vi "test-Implicit-Model-Follower-Test1.vi"(8 "error in (no error)":errorcluster) -> (0 "error out":errorcluster, 3 "All tests passed":bool)   [LabVIEW 2019]
uses:
  <vilib>/Rock Robotics/WPI/ThirdParty/JAS_Junk/TrajLib/MatBuilder_Create.vi
  <vilib>/Rock Robotics/WPI/ThirdParty/JAS_Junk/TrajLib/LinearSystem_New.vi
  <vilib>/Rock Robotics/WPI/ThirdParty/JAS_Junk/TrajLib/MatrixHelper_Zero.vi
  <vilib>/Rock Robotics/WPI/ThirdParty/JAS_Junk/TrajLib/Discretization_DiscretizeAB.vi
  <vilib>/Analysis/baseanly.llb/A x B.vi
  <vilib>/Analysis/baseanly.llb/Real A x B.vi
  <vilib>/Rock Robotics/WPI/ThirdParty/JAS_Junk/TrajLib/MatrixHelper_CoerceSize.vi
  <vilib>/Rock Robotics/WPI/ThirdParty/JAS_Junk/TrajLib/Matrix_Exp.vi
  <vilib>/Rock Robotics/WPI/ThirdParty/JAS_Junk/TrajLib/Matrix_AssignBlock.vi
  <vilib>/Rock Robotics/WPI/ThirdParty/JAS_Junk/TrajLib/Matrix_ExtractFrom.vi
  <vilib>/Analysis/7linalg.llb/Matrix Exp.vi
  <vilib>/Analysis/7linalg.llb/Real Matrix Exp.vi
  <vilib>/Analysis/Matrix/Numeric/Multiply/Multiply.vi
  <vilib>/Analysis/Matrix/Numeric/Multiply/Multiply - RM,R.vi
  <vilib>/Analysis/Matrix/Numeric/Add/Add.vi
  <vilib>/Analysis/Matrix/Numeric/Add/Add - RM,RM.vi
  <vilib>/Rock Robotics/WPI/ThirdParty/JAS_Junk/TrajLib/Trajectory_Library.lvlib
panel:
  out "Test 3":bool
  out "Test 2":bool
  out "Test 1":bool
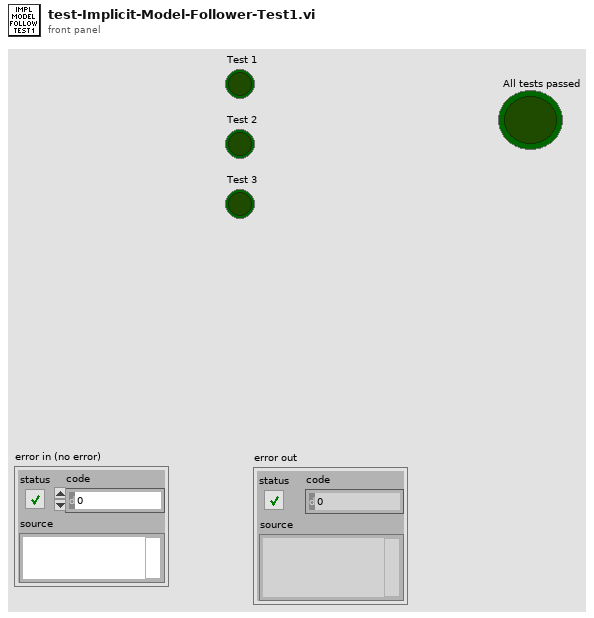
[diagram p1: front panel]
types:
  T1 = typedef "NI_Matrix.lvlib/RealMatrix.ctl" = dbl[][]
  T2 = typedef "Trajectory_Library.lvlib/LINEAR_SYSTEM.ctl" = cluster{"m_A":T1, "m_B":T1, "m_C":T1, "m_D":T1, "States":i32, "Inputs":i32, "Outputs":i32}
  T3 = typedef "Trajectory_Library.lvlib/IMPLICIT_MODEL_FOLLOWER.ctl" = cluster{"m_A":T1, "m_B":T1, "m_U":T1, "States":i32, "Inputs":i32}
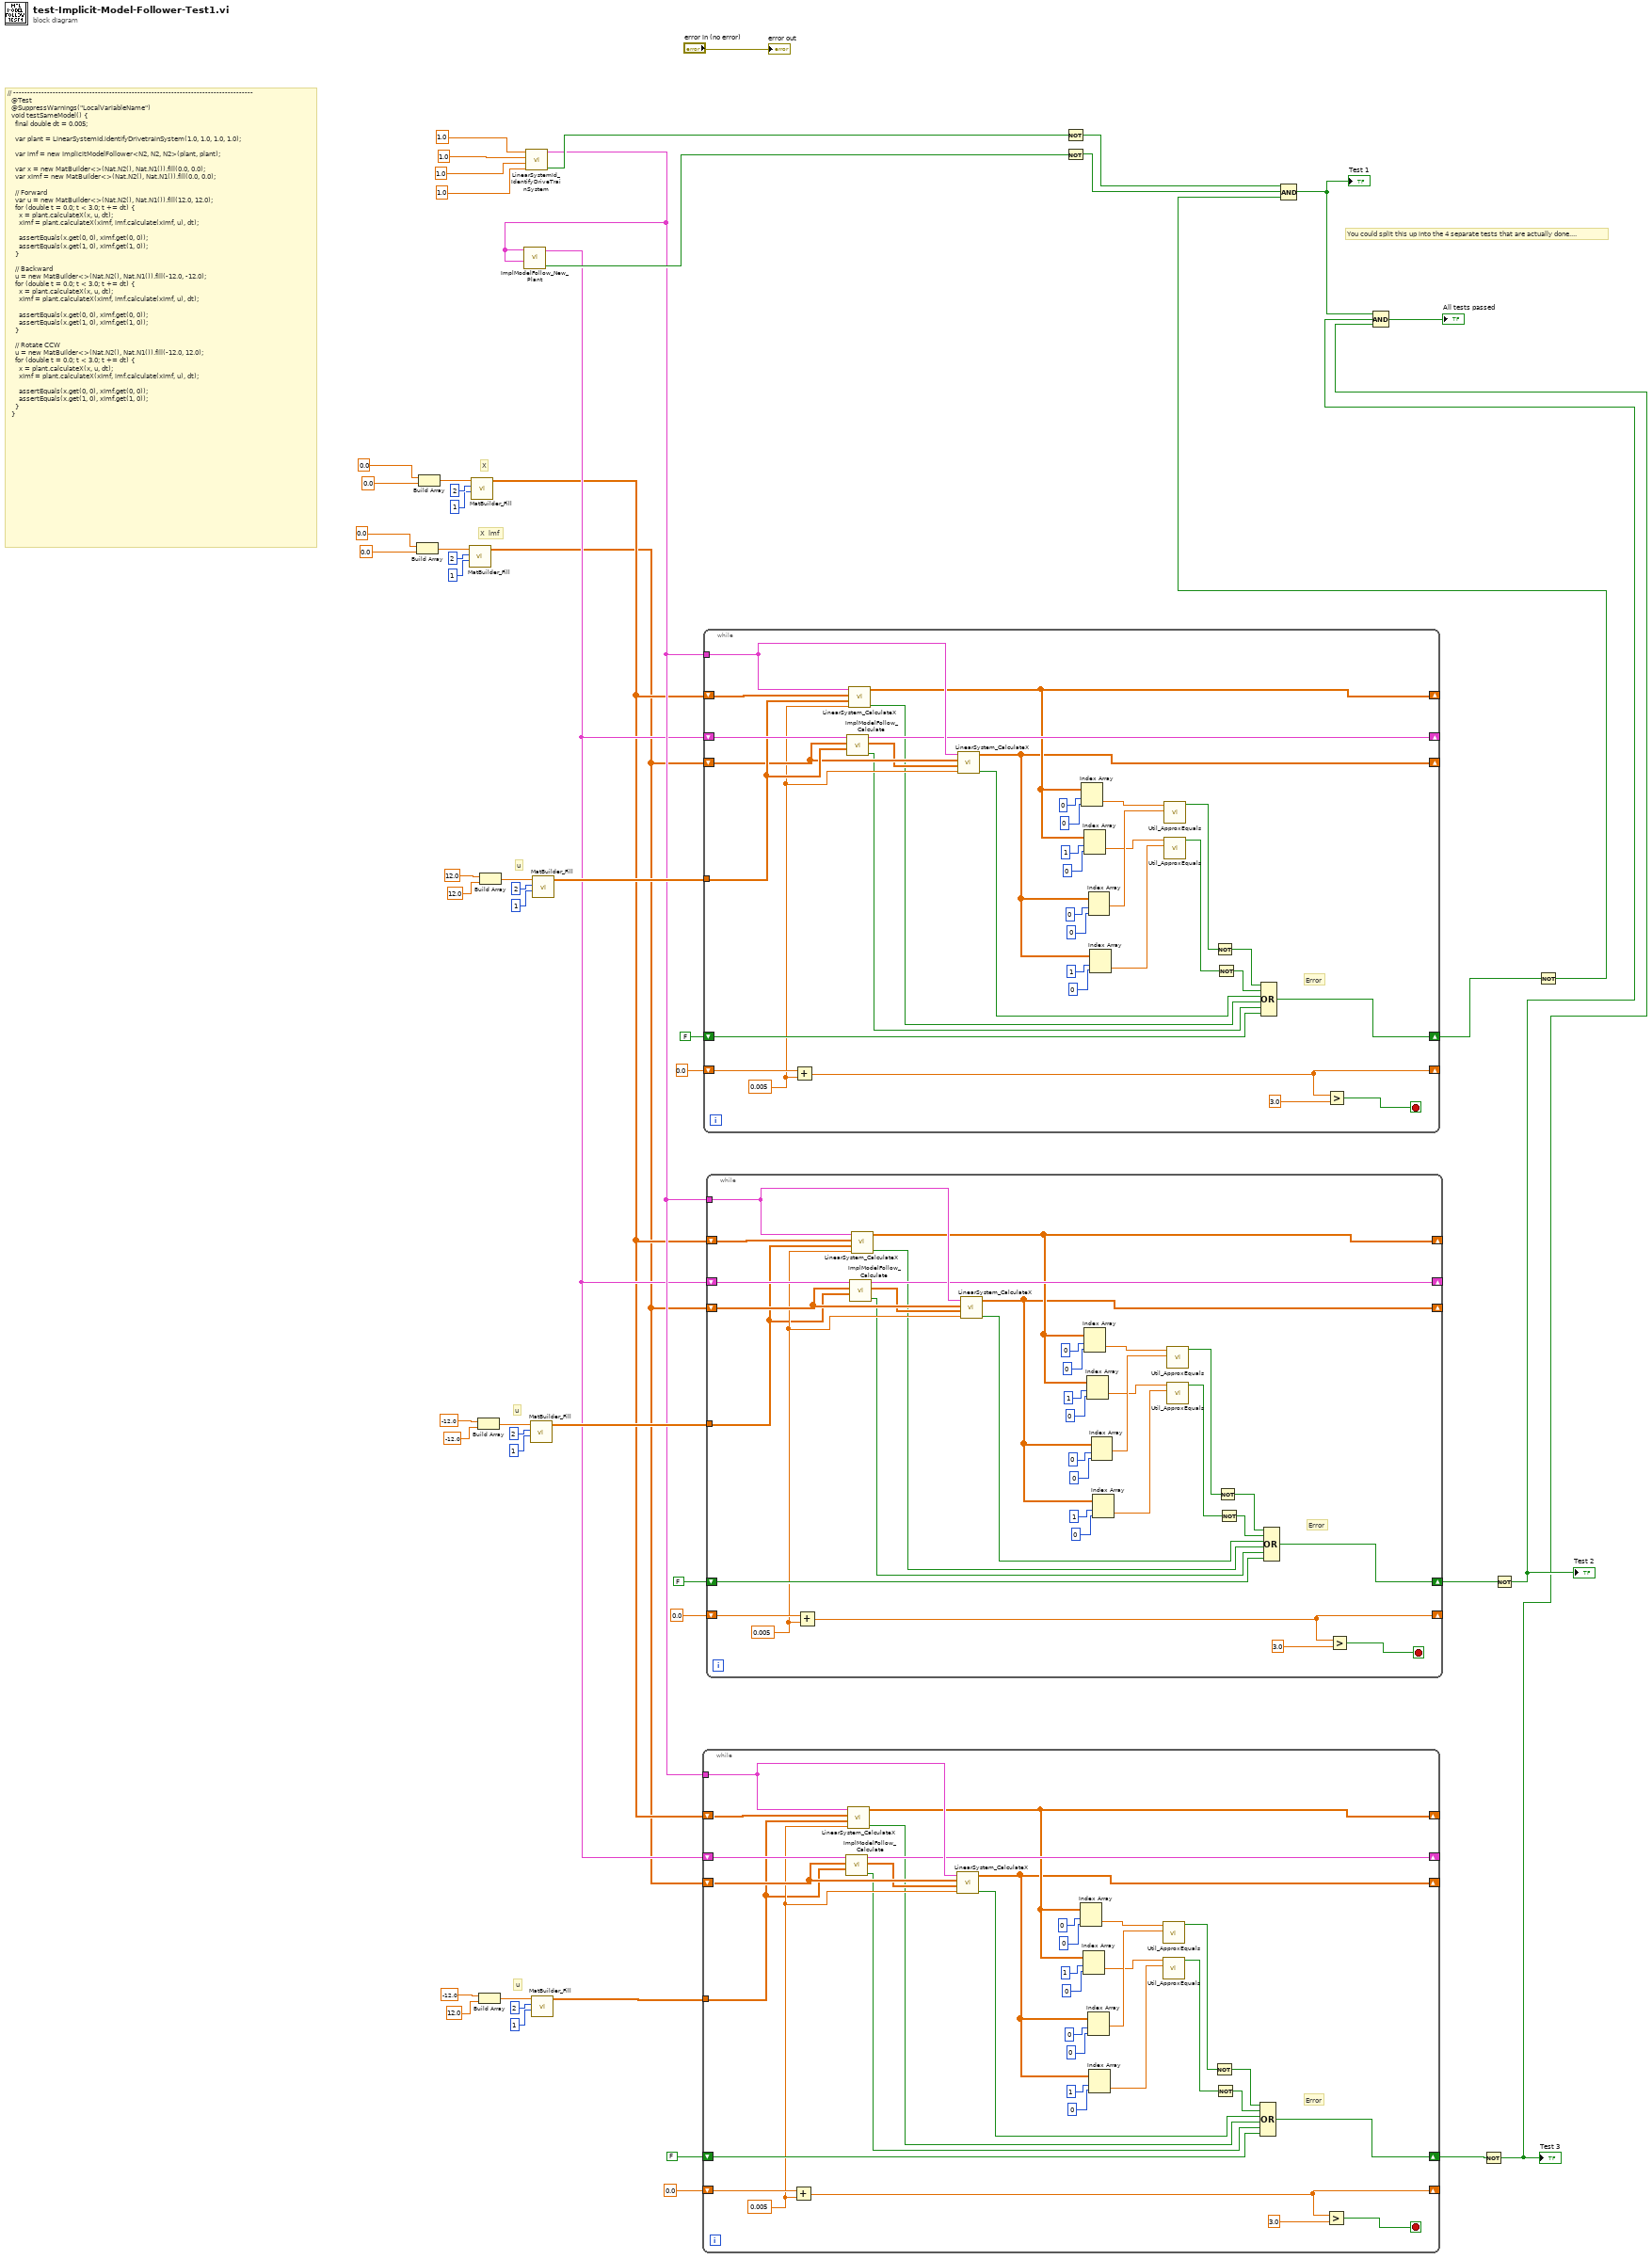
[diagram p0: block diagram]
diagram:
  # "X  lmf"
  # "// -------------------------------------------------------------------------------------\n  @Test\n  @SuppressWarnings(\"LocalVariableName\")\n  void testSameModel() {\n    final double dt = 0.005;\n\n    var plant = LinearSystemId.identifyDrivetrainSystem(1.0, 1.0, 1.0, 1.0);\n\n    var imf = new ImplicitModelFollower<N2, N2, N2>(plant, plant);\n\n    var x = new MatBuilder<>(Nat.N2(), Nat.N1()).fill(0.0, 0.0);\n    var xImf = new MatBuilder<>(Nat.N2(), Nat.N1()).fill(0.0, 0.0);\n\n    // Forward\n    var u = new MatBuilder<>(Nat.N2(), Nat.N1()).fill(12.0, 12.0);\n    for (double t = 0.0; t < 3.0; t += dt) {\n      x = plant.calculateX(x, u, dt);\n      xImf = plant.calculateX(xImf, imf.calculate(xImf, u), dt);\n\n      assertEquals(x.get(0, 0), xImf.get(0, 0));\n      assertEquals(x.get(1, 0), xImf.get(1, 0));\n    }\n\n    // Backward\n    u = new MatBuilder<>(Nat.N2(), Nat.N1()).fill(-12.0, -12.0);\n    for (double t = 0.0; t < 3.0; t += dt) {\n      x = plant.calculateX(x, u, dt);\n      xImf = plant.calculateX(xImf, imf.calculate(xImf, u), dt);\n\n      assertEquals(x.get(0, 0), xImf.get(0, 0));\n      assertEquals(x.get(1, 0), xImf.get(1, 0));\n    }\n\n    // Rotate CCW\n    u = new MatBuilder<>(Nat.N2(), Nat.N1()).fill(-12.0, 12.0);\n    for (double t = 0.0; t < 3.0; t += dt) {\n      x = plant.calculateX(x, u, dt);\n      xImf = plant.calculateX(xImf, imf.calculate(xImf, u), dt);\n\n      assertEquals(x.get(0, 0), xImf.get(0, 0));\n      assertEquals(x.get(1, 0), xImf.get(1, 0));\n    }\n  }"
  # "You could split this up into the 4 separate tests that are actually done...."
  # "u"
  # "u"
  # "u"
  # "X"
  n1 = Build Array(0.0 ("element"), 0.0 ("element")) -> (w24:dbl[])
  n2 = Build Array(0.0 ("element"), 0.0 ("element")) -> (w50:dbl[])
  n3 = call <vilib>:"MatBuilder_Fill.vi"("Columns"=1, "Rows"=2, "Value List"=w24) -> ("output matrix"=w4:T1)  [unwired: 8 in]
  n4 = call <vilib>:"MatBuilder_Fill.vi"("Columns"=1, "Rows"=2, "Value List"=w50) -> ("output matrix"=w5:T1)  [unwired: 8 in]
  n5 = Build Array(-12.0 ("element"), -12.0 ("element")) -> (w34:dbl[])
  n6 = Build Array(-12.0 ("element"), 12.0 ("element")) -> (w29:dbl[])
  n7 = Build Array(12.0 ("element"), 12.0 ("element")) -> (w44:dbl[])
  n8 = call <vilib>:"LinearSystemId_IdentifyDriveTrainSystem.vi"("kAAngular"=1.0 ("rbMeters"), "kVAngular"=1.0 ("rMeters"), "kALinear"=1.0 ("MassKg"), "kVLinear"=1.0 ("JKgMetersSquared")) -> ("Size Coerced"=w45:bool, "Linearsystem"=w7:T2)  [unwired: 6 in]
  n9 = call <vilib>:"ImplModelFollow_New_Plant.vi"("PlantRef"=w7, "Plant"=w7) -> ("Error"=w19:bool, "IMPLICIT_MODEL_FOLLOWER"=w6:T3)  [unwired: 8 in]
  n10 = call <vilib>:"MatBuilder_Fill.vi"("Columns"=1, "Rows"=2, "Value List"=w34) -> ("output matrix"=w12:T1)  [unwired: 8 in]
  n11 = call <vilib>:"MatBuilder_Fill.vi"("Columns"=1, "Rows"=2, "Value List"=w29) -> ("output matrix"=w8:T1)  [unwired: 8 in]
  n12 = call <vilib>:"MatBuilder_Fill.vi"("Columns"=1, "Rows"=2, "Value List"=w44) -> ("output matrix"=w38:T1)  [unwired: 8 in]
  n13 = while {
    shift-right: [w87] -> _
    shift-left: 0.0 -> [w90]
    tunnel: w7 -> [w77]
    shift-right: [w66] -> _
    shift-left: w5 -> [w86]
    shift-right: [w74] -> w1
    shift-left: FALSE -> [w75]
    shift-right: [w65] -> _
    shift-left: w4 -> [w71]
    shift-right: [w72] -> _
    shift-left: w6 -> [w73]
    tunnel: w8 -> [w56]
    stop <- w89 stop-if-true
    w69 = 0.005
    # "Error"
    n14 = Add(x=w90, y=w69) -> (x+y=w87:dbl)
    n15 = call <vilib>:"ImplModelFollow_Calculate.vi"("U"=w56, "X"=w71, "in IMPLICIT_MODEL_FOLLOWER"=w73) -> ("Error"=w67:bool, "U Out"=w70:T1, "out IMPLICIT_MODEL_FOLLOWER"=w72:T3)  [unwired: 6 in]
    n16 = call <vilib>:"LinearSystem_CalculateX.vi"("dT_Seconds"=w69, "ClampedU"=w56, "X"=w86, "Linearsystem"=w77) -> ("Error"=w68:bool, "outX"=w66:T1)  [unwired: 6 in]
    n17 = call <vilib>:"LinearSystem_CalculateX.vi"("dT_Seconds"=w69, "ClampedU"=w70, "X"=w71, "Linearsystem"=w77) -> ("Error"=w76:bool, "outX"=w65:T1)  [unwired: 6 in]
    n18 = Index Array(array=w66, index (row)=0, index (col)=0) -> (element=w64:dbl)
    n19 = Index Array(array=w66, index (row)=1, index (col)=0) -> (element=w62:dbl)
    n20 = Index Array(array=w65, index (row)=0, index (col)=0) -> (element=w63:dbl)
    n21 = Index Array(array=w65, index (row)=1, index (col)=0) -> (element=w61:dbl)
    n22 = call <vilib>:"Util_ApproxEquals.vi"("Value 2"=w63, "Value 1"=w64) -> ("ApproxEquals"=w58:bool)  [unwired: 9 in]
    n23 = call <vilib>:"Util_ApproxEquals.vi"("Value 2"=w61, "Value 1"=w62) -> ("ApproxEquals"=w57:bool)  [unwired: 9 in]
    n24 = Not(x=w58) -> (.not. x?=w59:bool)
    n25 = Not(x=w57) -> (.not. x?=w60:bool)
    n26 = Compound Arithmetic op=OR(w59, w60, w76, w68, w67, w75) -> (w74:bool)
    n27 = Greater?(x=w87, y=3.0) -> (0:w89:bool)
  }
  n28 = while {
    shift-right: [w122] -> _
    shift-left: 0.0 -> [w125]
    tunnel: w7 -> [w112]
    tunnel: w38 -> [w107]
    shift-right: [w100] -> _
    shift-left: w5 -> [w121]
    shift-right: [w109] -> w36
    shift-left: FALSE -> [w110]
    shift-right: [w99] -> _
    shift-left: w4 -> [w105]
    shift-right: [w106] -> _
    shift-left: w6 -> [w108]
    stop <- w124 stop-if-true
    w103 = 0.005
    # "Error"
    n29 = Add(x=w125, y=w103) -> (x+y=w122:dbl)
    n30 = call <vilib>:"ImplModelFollow_Calculate.vi"("U"=w107, "X"=w105, "in IMPLICIT_MODEL_FOLLOWER"=w108) -> ("Error"=w101:bool, "U Out"=w104:T1, "out IMPLICIT_MODEL_FOLLOWER"=w106:T3)  [unwired: 6 in]
    n31 = call <vilib>:"LinearSystem_CalculateX.vi"("dT_Seconds"=w103, "ClampedU"=w107, "X"=w121, "Linearsystem"=w112) -> ("Error"=w102:bool, "outX"=w100:T1)  [unwired: 6 in]
    n32 = call <vilib>:"LinearSystem_CalculateX.vi"("dT_Seconds"=w103, "ClampedU"=w104, "X"=w105, "Linearsystem"=w112) -> ("Error"=w111:bool, "outX"=w99:T1)  [unwired: 6 in]
    n33 = Index Array(array=w100, index (row)=0, index (col)=0) -> (element=w98:dbl)
    n34 = Index Array(array=w100, index (row)=1, index (col)=0) -> (element=w96:dbl)
    n35 = Index Array(array=w99, index (row)=0, index (col)=0) -> (element=w97:dbl)
    n36 = Index Array(array=w99, index (row)=1, index (col)=0) -> (element=w95:dbl)
    n37 = call <vilib>:"Util_ApproxEquals.vi"("Value 2"=w97, "Value 1"=w98) -> ("ApproxEquals"=w92:bool)  [unwired: 9 in]
    n38 = call <vilib>:"Util_ApproxEquals.vi"("Value 2"=w95, "Value 1"=w96) -> ("ApproxEquals"=w91:bool)  [unwired: 9 in]
    n39 = Not(x=w92) -> (.not. x?=w93:bool)
    n40 = Not(x=w91) -> (.not. x?=w94:bool)
    n41 = Compound Arithmetic op=OR(w93, w94, w111, w102, w101, w110) -> (w109:bool)
    n42 = Greater?(x=w122, y=3.0) -> (0:w124:bool)
  }
  n43 = while {
    shift-right: [w157] -> _
    shift-left: 0.0 -> [w160]
    tunnel: w7 -> [w147]
    shift-right: [w136] -> _
    shift-left: w5 -> [w156]
    shift-right: [w144] -> w9
    shift-left: FALSE -> [w145]
    shift-right: [w135] -> _
    shift-left: w4 -> [w141]
    shift-right: [w142] -> _
    shift-left: w6 -> [w143]
    tunnel: w12 -> [w126]
    stop <- w159 stop-if-true
    w139 = 0.005
    # "Error"
    n44 = Add(x=w160, y=w139) -> (x+y=w157:dbl)
    n45 = call <vilib>:"ImplModelFollow_Calculate.vi"("U"=w126, "X"=w141, "in IMPLICIT_MODEL_FOLLOWER"=w143) -> ("Error"=w137:bool, "U Out"=w140:T1, "out IMPLICIT_MODEL_FOLLOWER"=w142:T3)  [unwired: 6 in]
    n46 = call <vilib>:"LinearSystem_CalculateX.vi"("dT_Seconds"=w139, "ClampedU"=w126, "X"=w156, "Linearsystem"=w147) -> ("Error"=w138:bool, "outX"=w136:T1)  [unwired: 6 in]
    n47 = call <vilib>:"LinearSystem_CalculateX.vi"("dT_Seconds"=w139, "ClampedU"=w140, "X"=w141, "Linearsystem"=w147) -> ("Error"=w146:bool, "outX"=w135:T1)  [unwired: 6 in]
    n48 = Index Array(array=w136, index (row)=0, index (col)=0) -> (element=w134:dbl)
    n49 = Index Array(array=w136, index (row)=1, index (col)=0) -> (element=w132:dbl)
    n50 = Index Array(array=w135, index (row)=0, index (col)=0) -> (element=w133:dbl)
    n51 = Index Array(array=w135, index (row)=1, index (col)=0) -> (element=w131:dbl)
    n52 = call <vilib>:"Util_ApproxEquals.vi"("Value 2"=w133, "Value 1"=w134) -> ("ApproxEquals"=w128:bool)  [unwired: 9 in]
    n53 = call <vilib>:"Util_ApproxEquals.vi"("Value 2"=w131, "Value 1"=w132) -> ("ApproxEquals"=w127:bool)  [unwired: 9 in]
    n54 = Not(x=w128) -> (.not. x?=w129:bool)
    n55 = Not(x=w127) -> (.not. x?=w130:bool)
    n56 = Compound Arithmetic op=OR(w129, w130, w146, w138, w137, w145) -> (w144:bool)
    n57 = Greater?(x=w157, y=3.0) -> (0:w159:bool)
  }
  n58 = Not(x=w45) -> (.not. x?=w17:bool)
  n59 = Not(x=w19) -> (.not. x?=w18:bool)
  n60 = Not(x=w1) -> (.not. x?=w13:bool)
  "Test 3" <- w13
  n61 = Not(x=w9) -> (.not. x?=w14:bool)
  "Test 2" <- w14
  n62 = Not(x=w36) -> (.not. x?=w35:bool)
  n63 = Compound Arithmetic op=AND(w17, w18, w35) -> (w16:bool)
  "Test 1" <- w16
  n64 = Compound Arithmetic op=AND(w16, w14, w13) -> (→"All tests passed":bool)
  "error out" <- "error in (no error)"
